vi "Read Children Items.vi"(10 "Tag In":string, 11 "Tree in":refnum<class "Tree.lvclass">) -> (0 "Children Tag":string[](array[string]), 2 "Children Items":T1[](array[typedef]), 3 "Tree out":refnum<class "Tree.lvclass">)   [LabVIEW 2024, in "Tree.lvclass"]
doc: "Search the child items, if the input tag is empty string, \ntreat the first tag of all tags as the child tag."
uses:
  Tree.lvclass
  Type Def/Tree Item.ctl
  Tree.lvclass/Tree.ctl
  Polymorphic VIs/Tree Converter/Tag To BFS Index.vi
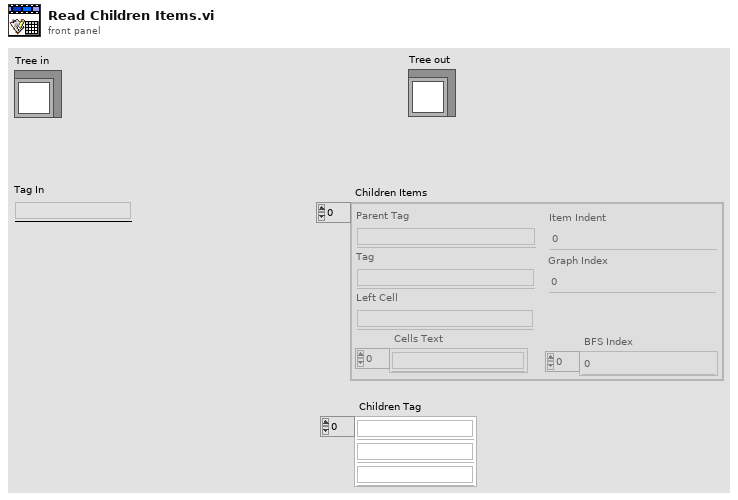
[diagram p1: front panel]
types:
  T1 = typedef "Tree Item.ctl" = cluster{"Parent Tag":string, "Tag":string, "Left Cell":string, "Cells Text":string[], "BFS Index":i32[], "Graph Index":i32, "Item Indent":i32}
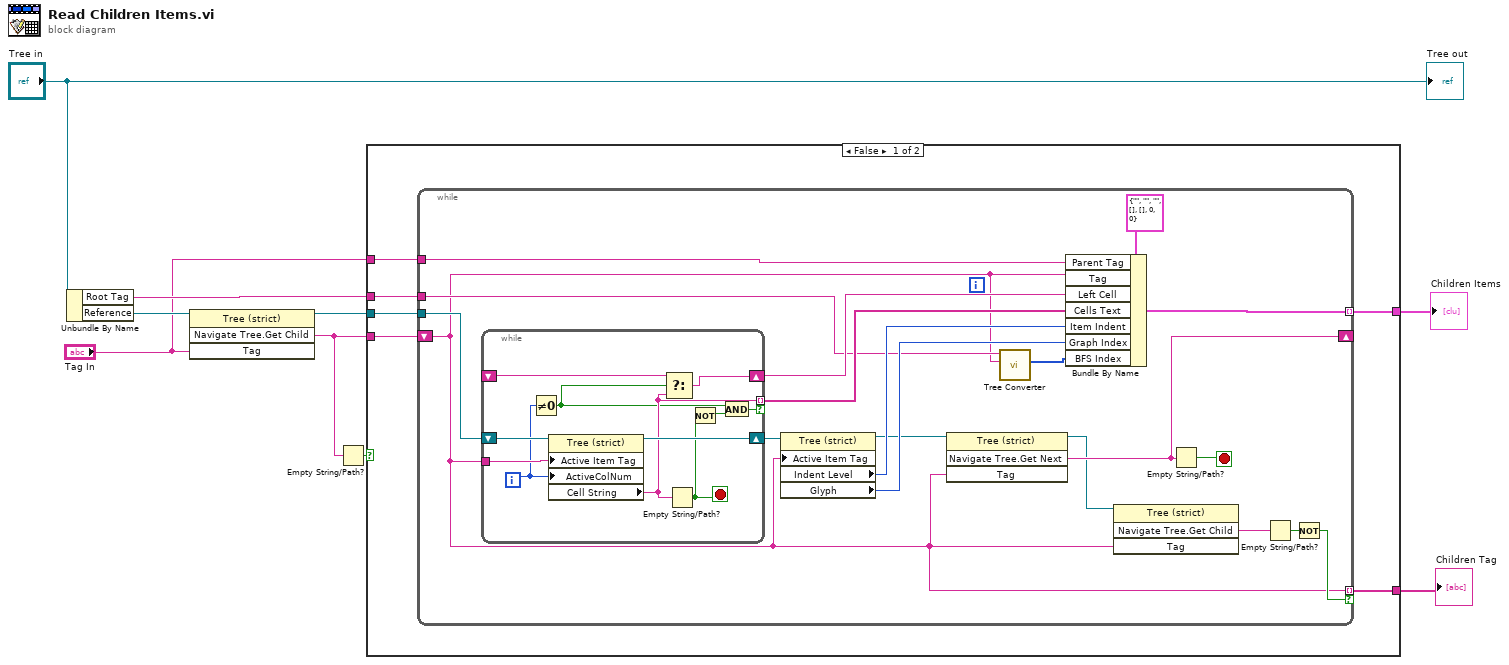
[diagram p0: block diagram]
diagram:
  n1 = Unbundle By Name("Tree in") -> ("Root Tag"=w4:string, "Reference"=w9:refnum<vi>)
  n2 = invoke class="Tree (strict)" method="Navigate Tree.Get Child"(reference=w9, "Tag"="Tag In") -> (reference out=w7:refnum<vi>, "Navigate Tree:Get Child"=w5:string)  [unwired: 2 in, 2 out]
  n3 = Empty String/Path?(string/path=w5) -> (empty?=w6:bool)
  n4 = case shown="False" w6 {
    tunnel: w5 -> [w15 _]
    tunnel: w7 -> [w14 _]
    tunnel: "Tag In" -> [w13 _]
    tunnel: [w12 _] -> w1
    tunnel: [w11 _] -> w2
    tunnel: w4 -> [w10 _]
    frame False {
      n5 = while {
        tunnel: [w28] -> w11 mode=indexing
        tunnel: w14 -> [w27]
        shift-right: [w24] -> _
        shift-left: w15 -> [w16]
        tunnel: w13 -> [w26]
        tunnel: [w16] -> w12 mode=indexing if=w19
        tunnel: w10 -> [w17]
        stop <- w23 stop-if-true
        n6 = while {
          tunnel: w16 -> [w44]
          shift-right: [w43] -> w31
          shift-left: w27 -> [w45]
          tunnel: [w41] -> w33 mode=indexing if=w37
          shift-right: [w40] -> w32
          shift-left: _ -> [w39]
          i -> [w42]
          stop <- w35 stop-if-true
          n7 = Not Equal To 0?(x=w42) -> (x != 0?=w38:bool)
          n8 = property class="Tree (strict)"(reference=w45, "Active Item Tag"=w44, "ActiveColNum"=w42) -> (reference out=w43:refnum<vi>, "Cell String"=w41:string)  [unwired: 1 in, 1 out]
          n9 = Select(t=w39, s=w38, f=w41) -> (s? t:f=w40:string)
          n10 = Empty String/Path?(string/path=w41) -> (empty?=w35:bool)
          n11 = Not(x=w35) -> (.not. x?=w36:bool)
          n12 = And(x=w38, y=w36) -> (x .and. y?=w37:bool)
        }
        n13 = property class="Tree (strict)"(reference=w31, "Active Item Tag"=w16) -> (reference out=w25:refnum<vi>, "Indent Level"=w30:i32, "Glyph"=w29:i32)  [unwired: 1 in, 1 out]
        n14 = invoke class="Tree (strict)" method="Navigate Tree.Get Next"(reference=w25, "Tag"=w16) -> (reference out=w22:refnum<vi>, "Navigate Tree:Get Next Item"=w24:string)  [unwired: 2 in, 2 out]
        n15 = call-poly "Tree Converter.vi"("Tag In"=w16, "Root Tag"=w17) -> ("BFS Index Out"=w18:i32[])  [unwired: 9 in]
        n16 = Bundle By Name(cluster=T1 {"Parent Tag"="", "Tag"="", "Left Cell"="", "Cells Text"=[], "BFS Index"=[], "Graph Index"=0, "Item Indent"=0} ("TreeItem"), "Parent Tag"=w26, "Tag"=w16, "Left Cell"=w32, "Cells Text"=w33, "Item Indent"=w30, "Graph Index"=w29, "BFS Index"=w18) -> (w28:T1)
        n17 = invoke class="Tree (strict)" method="Navigate Tree.Get Child"(reference=w22, "Tag"=w16) -> ("Navigate Tree:Get Child"=w21:string)  [unwired: 2 in, 3 out]
        n18 = Empty String/Path?(string/path=w24) -> (empty?=w23:bool)
        n19 = Empty String/Path?(string/path=w21) -> (empty?=w20:bool)
        n20 = Not(x=w20) -> (.not. x?=w19:bool)
      }
    }
    frame True {
    }
  }
  "Children Items" <- w2
  "Children Tag" <- w1
  "Tree out" <- "Tree in"
